vi "Write IO Configuration File.vi"(8 "error in (no error)":errorcluster, 10 "IO Nodes":T1 {"AO Config"."AO Channels"."Conversion"."ScaleOffset" format="%.3f"; "AO Config"."AO Channels"."Conversion"."MinEngUnit" format="%.3f"; "AO Config"."AO Channels"."Conversion"."MaxEngUnit" format="%.3f"; "AO Config"."AO Channels"."Conversion"."MinSignal" format="%.3f"; "AO Config"."AO Channels"."Conversion"."MaxSignal" format="%.3f"; "AI Config"."AI Tasks"."AI Channels"."Conversion"."ScaleOffset" format="%.3f"; "AI Config"."AI Tasks"."AI Channels"."Conversion"."MinEngUnit" format="%.3f"; "AI Config"."AI Tasks"."AI Channels"."Conversion"."MaxEngUnit" format="%.3f"; "AI Config"."AI Tasks"."AI Channels"."Conversion"."MinSignal" format="%.3f"; "AI Config"."AI Tasks"."AI Channels"."Conversion"."MaxSignal" format="%.3f"; "AI Config"."AI Tasks"."AI Channels"."Terminal Configuration" items=["default"=-1, "RSE"=10083, "NRSE"=10078, "Differential"=10106, "Pseudodifferential"=12529]}, 11 "DAQ ConfigFile":path) -> (0 "error out":errorcluster)   [LabVIEW 2020, in "DAQ.lvclass"]
doc: "Developed by Kevin Thompson\nkevin@thompsonengineering.net\n\nCopyright 2015\nThompson Engineering, LLC\nWrites file: \"IOConfig.ini\" at \"ConfigFolder\" folder."
uses:
  DAQ.lvclass
  DAQ.lvclass/DAQ.ctl
  DataTypes/TD AI Channel--cluster.ctl
  DataTypes/TD AI Config--cluster.ctl
  DataTypes/TD AO Channel--cluster.ctl
  DataTypes/TD AO Config--cluster.ctl
  DataTypes/TD DI Channel--cluster.ctl
  DataTypes/TD DI Config--cluster.ctl
  DataTypes/TD DO Channel--cluster.ctl
  DataTypes/TD DO Config--cluster.ctl
  DataTypes/TD IO Node Definition--cluster.ctl
  DataTypes/TD DataValueConversion--cluster.ctl
  DataTypes/TD AI DAQ Type--enum.ctl
  DataTypes/TD AI Task--cluster.ctl
  DataTypes/TD DI Task--cluster.ctl
  DataTypes/TD AI Force Bridge--cluster.ctl
panel:
  # "Writes file: \"IOConfig.ini\"\nat \"ConfigFolder\" folder."
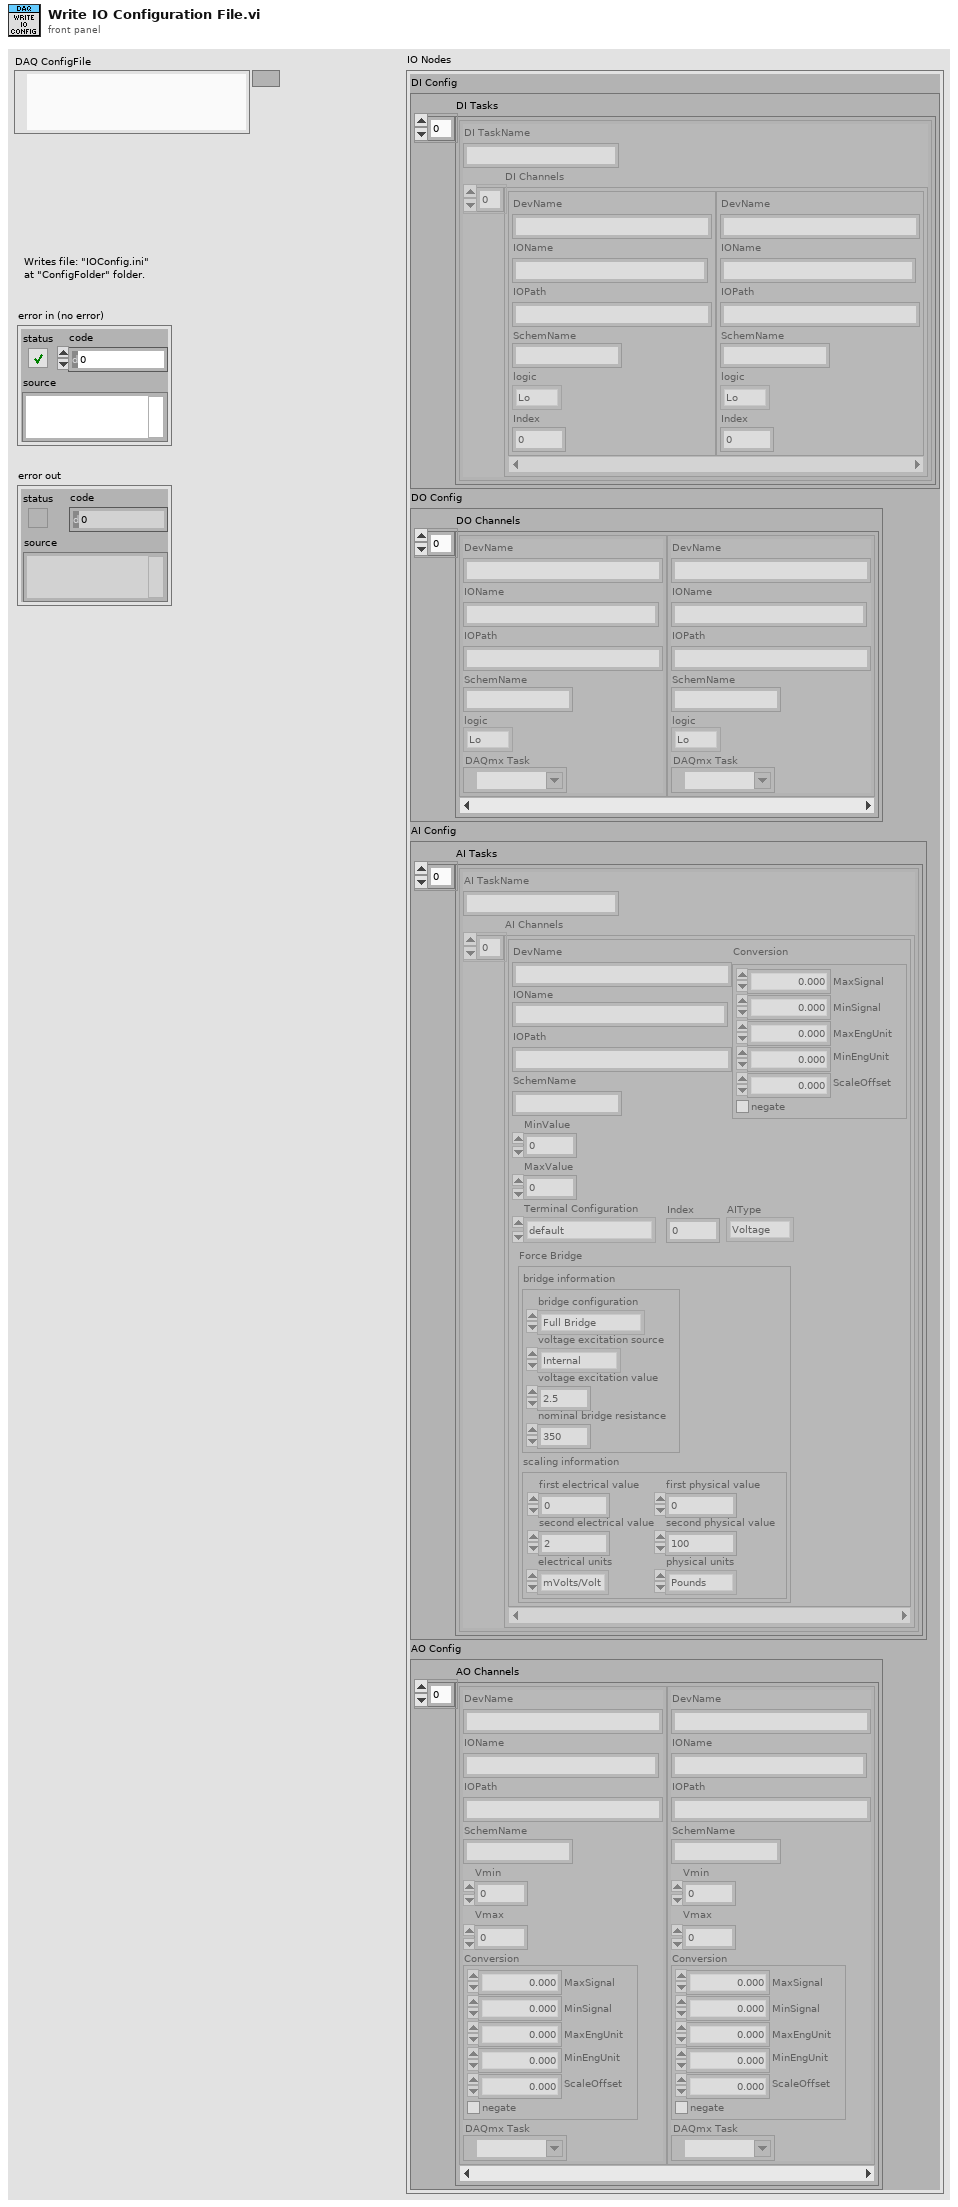
[diagram p1: front panel]
types:
  T1 = typedef "DAQ.lvclass/TD IO Node Definition--cluster.ctl" = cluster{"DI Config":T2, "DO Config":T5, "AI Config":T7, "AO Config":T13}
  T2 = typedef "DAQ.lvclass/TD DI Config--cluster.ctl" = cluster{"DI Tasks":T3[]}
  T3 = typedef "DAQ.lvclass/TD DI Task--cluster.ctl" = cluster{"DI TaskName":string, "DI Channels":T4[]}
  T4 = typedef "DAQ.lvclass/TD DI Channel--cluster.ctl" = cluster{"DevName":string, "IOName":string, "IOPath":string, "SchemName":string, "logic":enum16{"Lo", "Hi"}, "Index":i32}
  T5 = typedef "DAQ.lvclass/TD DO Config--cluster.ctl" = cluster{"DO Channels":T6[]}
  T6 = typedef "DAQ.lvclass/TD DO Channel--cluster.ctl" = cluster{"DevName":string, "IOName":string, "IOPath":string, "SchemName":string, "logic":enum16{"Lo", "Hi"}, "DAQmx Task":refnum<k21>}
  T7 = typedef "DAQ.lvclass/TD AI Config--cluster.ctl" = cluster{"AI Tasks":T8[]}
  T8 = typedef "DAQ.lvclass/TD AI Task--cluster.ctl" = cluster{"AI TaskName":string, "AI Channels":T9[]}
  T9 = typedef "DAQ.lvclass/TD AI Channel--cluster.ctl" = cluster{"DevName":string, "IOName":string, "IOPath":string, "SchemName":string, "MinValue":dbl, "MaxValue":dbl, "Terminal Configuration":i32, "Index":i32, "Conversion":T10, "AIType":T11, "Force Bridge":T12}
  T10 = typedef "DAQ.lvclass/TD DataValueConversion--cluster.ctl" = cluster{"MaxSignal":dbl, "MinSignal":dbl, "MaxEngUnit":dbl, "MinEngUnit":dbl, "ScaleOffset":dbl, "negate":bool}
  T11 = typedef "DAQ.lvclass/TD AI DAQ Type--enum.ctl" = enum16{"Voltage", "Current", "Strain Gage", "Force Bridge"}
  T12 = typedef "DAQ.lvclass/TD AI Force Bridge--cluster.ctl" = cluster{"bridge information":cluster{"bridge configuration":i32, "voltage excitation source":i32, "voltage excitation value":dbl, "nominal bridge resistance":dbl}, "scaling information":cluster{"first electrical value":dbl, "second electrical value":dbl, "electrical units":i32, "first physical value":dbl, "second physical value":dbl, "physical units":i32}}
  T13 = typedef "DAQ.lvclass/TD AO Config--cluster.ctl" = cluster{"AO Channels":T14[]}
  T14 = typedef "DAQ.lvclass/TD AO Channel--cluster.ctl" = cluster{"DevName":string, "IOName":string, "IOPath":string, "SchemName":string, "Vmin":dbl, "Vmax":dbl, "Conversion":T10, "DAQmx Task":refnum<k21>}
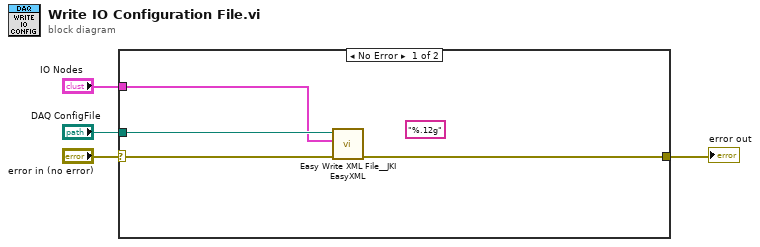
[diagram p0: block diagram]
diagram:
  n1 = case shown="No Error" "error in (no error)" {
    selector: "error in (no error)" -> [w8 w9]
    tunnel: "IO Nodes" -> [w6 _]
    tunnel: "DAQ ConfigFile" -> [w7 _]
    tunnel: [w5 w9] -> w2
    frame No Error {
      (unwired) "%.12g" ("float number format (optional)")
      n2 = call <vilib>:"Easy Write XML File__JKI EasyXML.vi"("error in (no error)"=w8, "LabVIEW Data"=w6, "XML File Path"=w7) -> ("error out"=w5:errorcluster)  [unwired: 7 in, 1 out]
    }
    frame Error {
    }
  }
  "error out" <- w2
